vi "V7001 Message Loop.vi"(8 "error in (no error)":errorcluster, 9 "Data Queue":refnum<queue>, 10 "Data Notifier":refnum<notifier>, 11 "Message Queues":T1) -> (0 "error out":errorcluster)   [LabVIEW 2015, in "V7001.lvlib"]
uses:
  V7001.lvlib
  support/Message Queue/All Message Queues.ctl
  support/Message Queue/Message Cluster.ctl
  V7001 Configuration.ctl
  V7001 State.ctl
  V7001 Loop State.ctl
  <vilib>/Utility/error.llb/Error Cluster From Error Code.vi
  <vilib>/ErrorRing/Error Ring.xnode
  support/Message Queue/Message Queue.lvlib
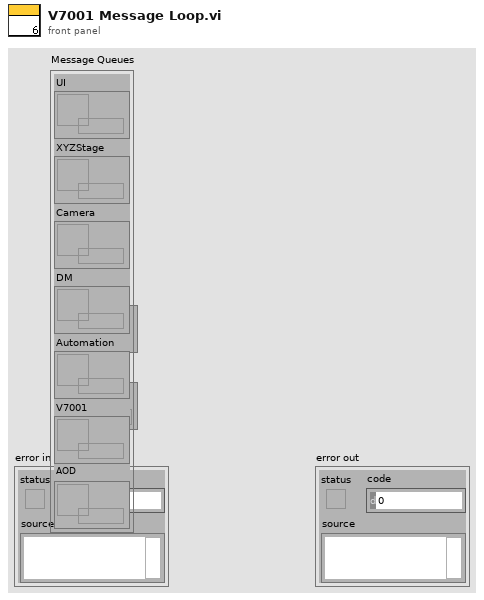
[diagram p1: front panel]
types:
  T1 = typedef "Message Queue.lvlib/All Message Queues.ctl" = cluster{"UI":refnum<queue>, "XYZStage":refnum<queue>, "Camera":refnum<queue>, "DM":refnum<queue>, "Automation":refnum<queue>, "V7001":refnum<queue>, "AOD":refnum<queue>}
  T2 = typedef "V7001.lvlib/V7001 State.ctl" = cluster{"V7001 State":T3, "Handle out":u32, "Size":dbl[]}
  T3 = typedef "V7001.lvlib/V7001 Loop State.ctl" = enum16{"Idle", "Connected"}
  T4 = typedef "V7001.lvlib/V7001 Configuration.ctl" = cluster{" Index":u32}
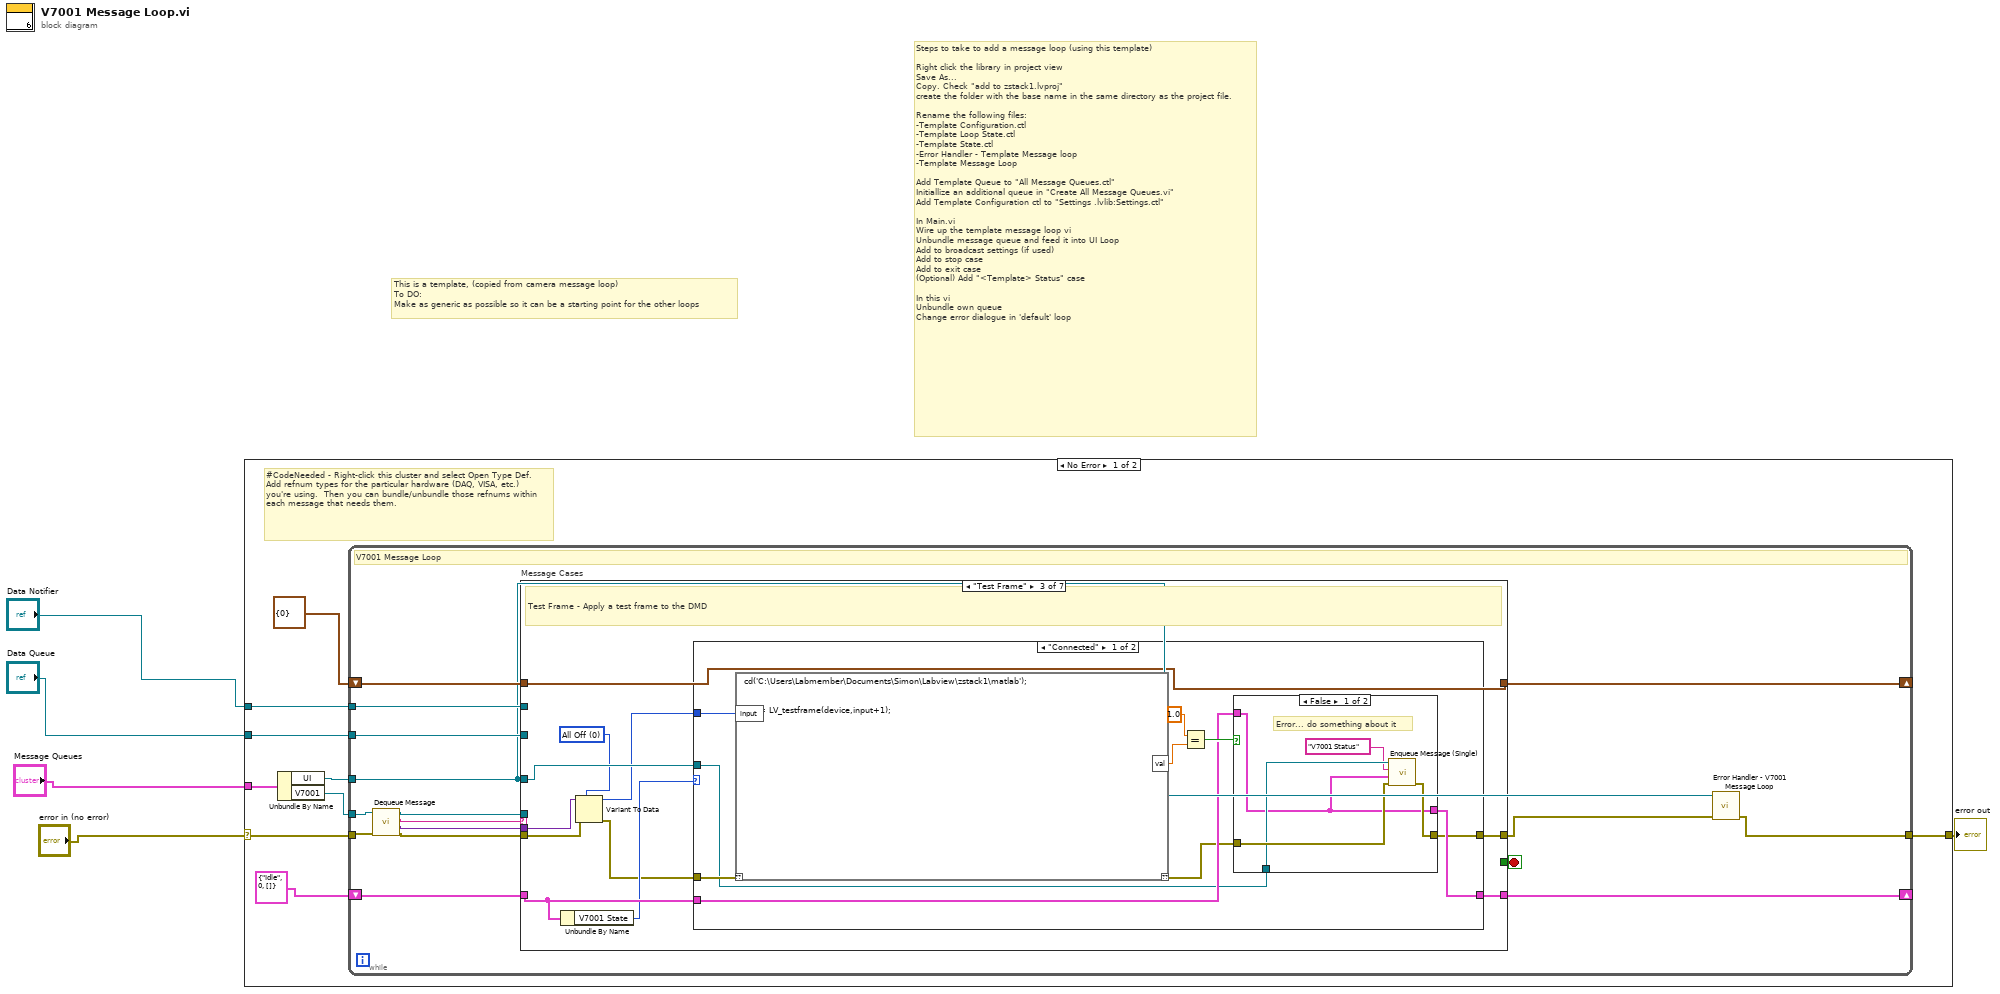
[diagram p0: block diagram]
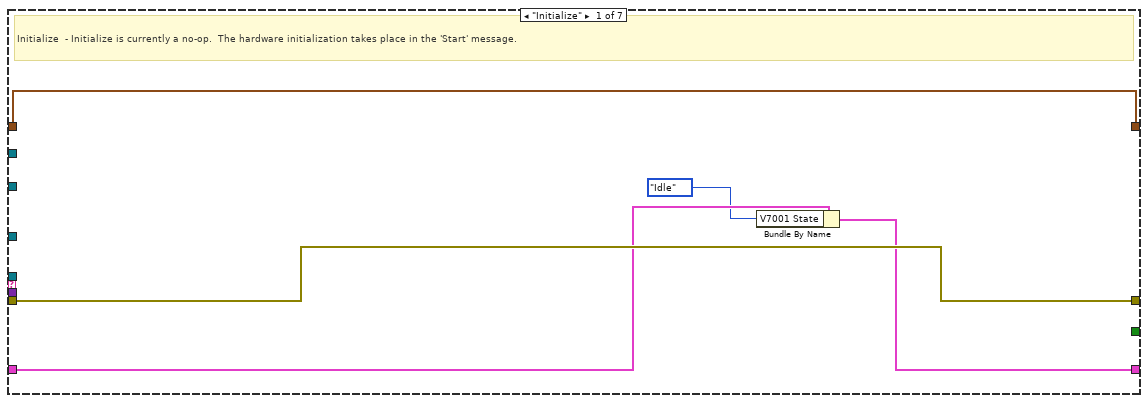
[diagram p2: hidden frame]
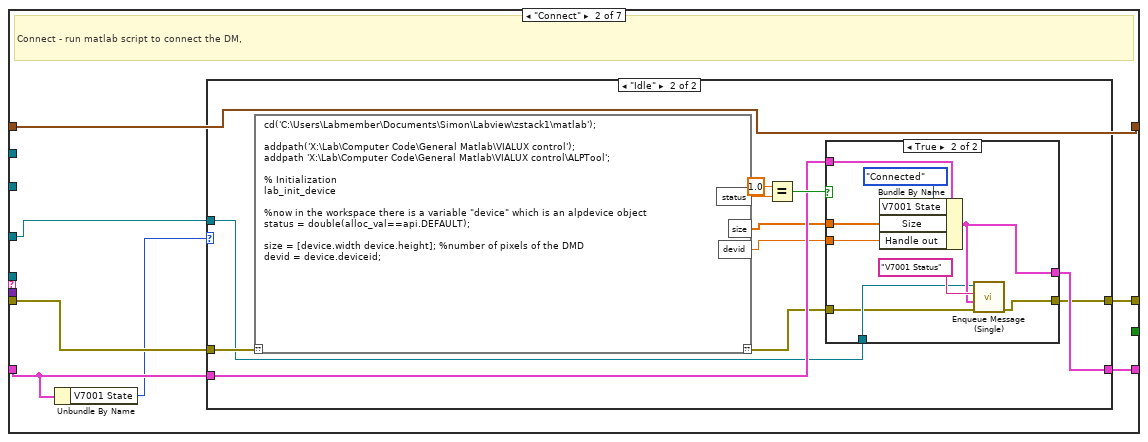
[diagram p3: hidden frame]
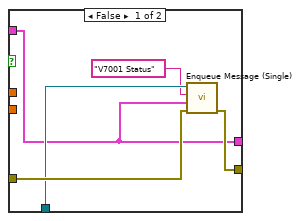
[diagram p5: hidden frame]
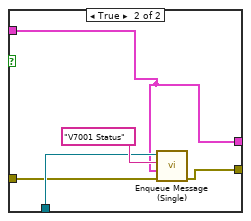
[diagram p6: hidden frame]
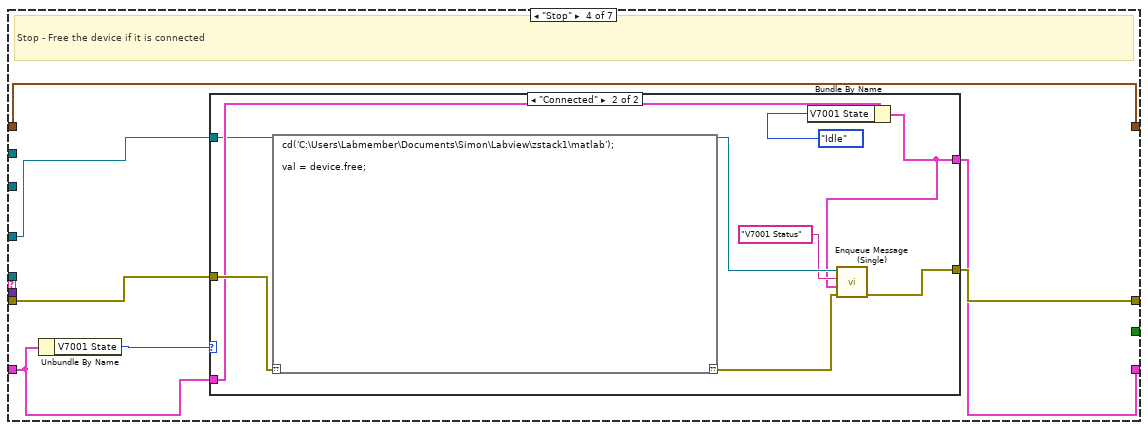
[diagram p8: hidden frame]
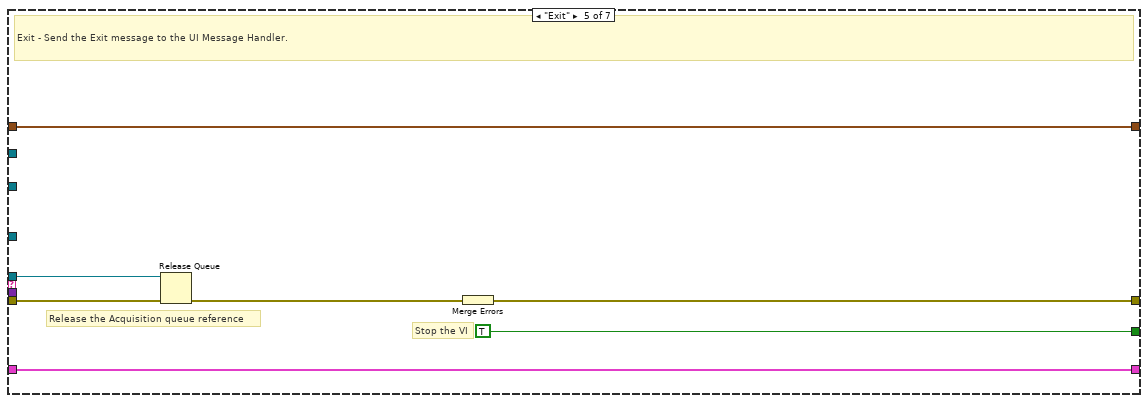
[diagram p10: hidden frame]
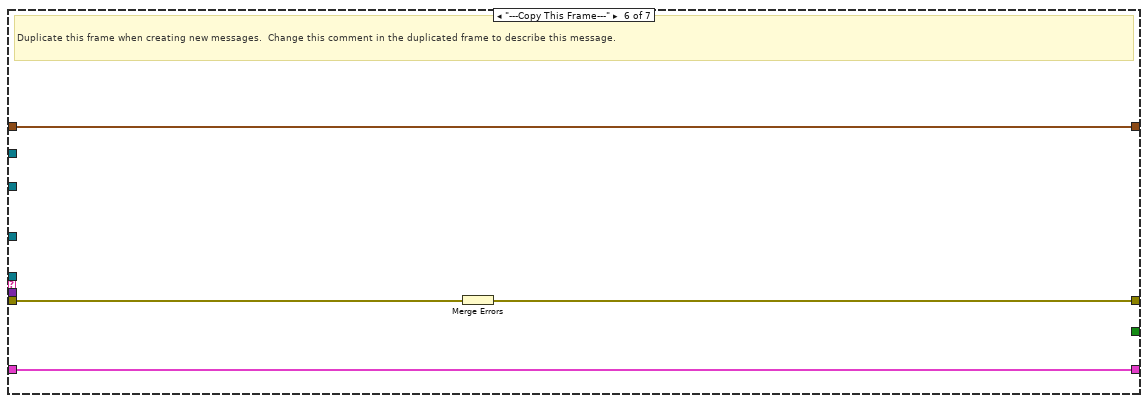
[diagram p11: hidden frame]
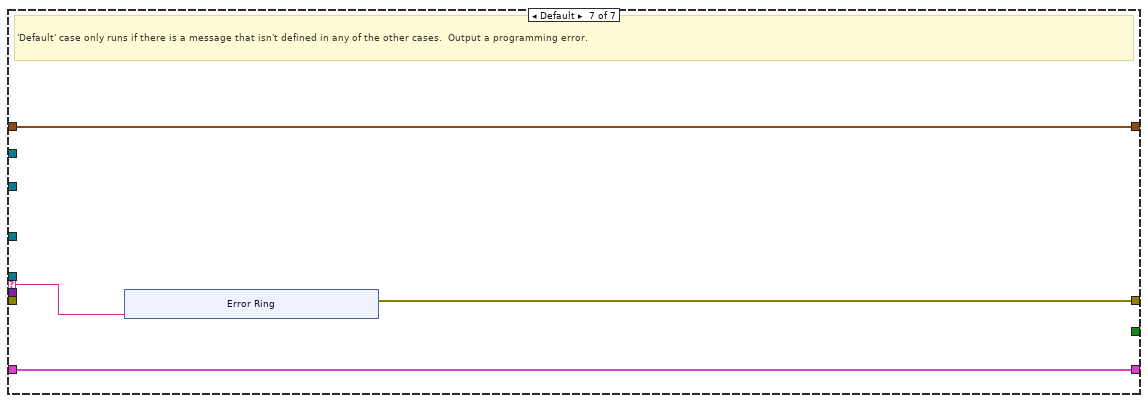
[diagram p12: hidden frame]
diagram:
  # "Steps to take to add a message loop (using this template)\n\nRight click the library in project view\nSave As...\nCopy. Check \"add to zstack1.lvproj\"\ncreate the folder with the base name in the same directory as the project file.\n\nRename the following files:\n-Template Configuration.ctl\n-Template Loop State.ctl\n-Template State.ctl\n-Error Handler - Template Message loop\n-Template Message Loop\n\nAdd Template Queue to \"All Message Queues.ctl\"\nInitiallize an additional queue in \"Create All Message Queues.vi\"\nAdd Template Configuration ctl to \"Settings .lvlib:Settings.ctl\"\n\nIn Main.vi\nWire up the template message loop vi\nUnbundle message queue and feed it into UI Loop\nAdd to broadcast settings (if used)\nAdd to stop case\nAdd to exit case\n(Optional) Add \"<Template> Status\" case\n\nIn this vi\nUnbundle own queue\nChange error dialogue in 'default' loop"
  # "This is a template, (copied from camera message loop)\nTo DO:\nMake as generic as possible so it can be a starting point for the other loops"
  n1 = case shown="No Error" "error in (no error)" {
    selector: "error in (no error)" -> [w11 w142]
    tunnel: "Message Queues" -> [w14 _]
    tunnel: [w12 w142] -> w5
    tunnel: "Data Notifier" -> [w9 _]
    tunnel: "Data Queue" -> [w8 _]
    frame No Error {
      # "#CodeNeeded - Right-click this cluster and select Open Type Def.  Add refnum types for the particular hardware (DAQ, VISA, etc.) you're using.  Then you can bundle/unbundle those refnums within each message that needs them."
      n2 = Unbundle By Name(w14) -> ("UI"=w10:refnum<queue>, "V7001"=w13:refnum<queue>)
      n3 = while {
        tunnel: w13 -> [w23]
        shift-right: [w29] -> _
        shift-left: T4 {" Index"=0} ("Hardware Configuration") -> [w30]
        tunnel: w10 -> [w15]
        tunnel: w9 -> [w27]
        tunnel: w8 -> [w26]
        shift-right: [w24] -> _
        shift-left: T2 {"V7001 State"=enum."Idle", "Handle out"=0, "Size"=[]} ("Cluster") -> [w25]
        tunnel: w11 -> [w22]
        tunnel: [w17] -> w12
        stop <- w28 stop-if-true
        # "V7001 Message Loop"
        n4 = call "Dequeue Message.vi"("error in (no error)"=w22, "Message Queue"=w23) -> ("error out"=w18:errorcluster, "Message Data"=w19:variant, "Message"=w20:string, "dup Message Queue"=w21:refnum<queue>)  [unwired: 6 in]
        n5 = case "Message Cases" shown="\"Test Frame\"" w20 {
          selector: w20 -> [_ _ _ _ _ _ w131]
          tunnel: w21 -> [_ _ _ _ w121 _ _]
          tunnel: w18 -> [w34 w41 w71 w107 w123 w130 _]
          tunnel: [w34 w36 w75 w106 w125 w128 w132] -> w16
          tunnel: w30 -> [w35 w42 w80 w109 w124 w129 w134]
          tunnel: [w35 w42 w80 w109 w124 w129 w134] -> w29
          tunnel: [_ _ _ _ TRUE _ _] -> w28
          tunnel: w19 -> [_ _ w74 _ _ _ _]
          tunnel: w15 -> [_ w37 w76 w103 _ _ _]
          tunnel: w27 -> [_ _ _ _ _ _ _]
          tunnel: w26 -> [_ _ _ _ _ _ _]
          tunnel: w25 -> [w32 w39 w78 w105 w120 w127 w133]
          tunnel: [w33 w40 w79 w104 w120 w127 w133] -> w24
          frame "Initialize" {
            # "Initialize  - Initialize is currently a no-op.  The hardware initialization takes place in the 'Start' message."
            n6 = Bundle By Name(cluster=w32, "V7001 State"=V7001_Loop_State."Idle") -> (w33:T2)
          }
          frame "Connect" {
            # "Connect - run matlab script to connect the DM,"
            n7 = Unbundle By Name(w39) -> ("V7001 State"=w38:T3)
            n8 = case shown="\"Idle\"" w38 {
              tunnel: w41 -> [w44 w55]
              tunnel: w39 -> [w43 w51]
              tunnel: [w43 w50] -> w40
              tunnel: w37 -> [_ w48]
              tunnel: [w44 w46] -> w36
              frame "Connected", Default {
              }
              frame "Idle" {
                n9 = script code="cd('C:\\Users\\Labmember\\Documents\\Simon\\Labview\\zstack1\\matlab');\n\naddpath('X:\\Lab\\Computer Code\\General Matlab\\VIALUX control');\naddpath 'X:\\Lab\\Computer Code\\General Matlab\\VIALUX control\\ALPTool';\n\n% Initialization \nlab_init_device\n\n%now in the workspace there is a variable \"device\" which is an alpdevice object\nstatus = double(alloc_val==api.DEFAULT);\n\nsize = [device.width device.height]; %number of pixels of the DMD\ndevid = device.deviceid;"("??"=w55) -> ("??"=w47:errorcluster, "status"=w54:dbl, "size"=w49:dbl[], "devid"=w45:dbl)
                n10 = Equal?(x=1.0, y=w54) -> (x = y?=w52:bool)
                n11 = case shown="True" w52 {
                  tunnel: [w56 w65] -> w50
                  tunnel: w51 -> [w56 w69]
                  tunnel: w49 -> [_ w67]
                  tunnel: w48 -> [w58 w64]
                  tunnel: w47 -> [w59 w63]
                  tunnel: [w60 w62] -> w46
                  tunnel: w45 -> [_ w61]
                  frame False {
                    n12 = call "Enqueue Message (Single).vi"("error in (no error)"=w59, "Message Data"=w56, "Message"="V7001 Status", "Message Queue"=w58) -> ("error out"=w60:errorcluster)  [unwired: 6 in, 1 out]
                  }
                  frame True {
                    n13 = Bundle By Name(cluster=w69, "V7001 State"=V7001_Loop_State."Connected", "Size"=w67, "Handle out"=w61) -> (w65:T2)
                    n14 = call "Enqueue Message (Single).vi"("error in (no error)"=w63, "Message Data"=w65, "Message"="V7001 Status", "Message Queue"=w64) -> ("error out"=w62:errorcluster)  [unwired: 6 in, 1 out]
                  }
                }
              }
            }
          }
          frame "Test Frame" {
            w73 = u16 0 items=["All Off", "All On", "Checkerboard 1", "Random"] ("Frame")
            # "Test Frame - Apply a test frame to the DMD"
            n15 = Unbundle By Name(w78) -> ("V7001 State"=w77:T3)
            n16 = Variant To Data(error in=w71, type=w73, Variant=w74) -> (data=w72:u16, error out=w70:errorcluster)
            n17 = case shown="\"Connected\"" w77 {
              tunnel: w70 -> [w90 w102]
              tunnel: w78 -> [w86 w101]
              tunnel: [w85 w101] -> w79
              tunnel: w76 -> [w84 _]
              tunnel: [w82 w102] -> w75
              tunnel: w72 -> [w81 _]
              frame "Connected" {
                n18 = script code="cd('C:\\Users\\Labmember\\Documents\\Simon\\Labview\\zstack1\\matlab');\n\n\nval = LV_testframe(device,input+1);"("??"=w90, "input"=w81) -> ("??"=w83:errorcluster, "val"=w89:dbl)
                n19 = Equal?(x=1.0, y=w89) -> (x = y?=w87:bool)
                n20 = case shown="False" w87 {
                  tunnel: [w91 w96] -> w85
                  tunnel: w86 -> [w91 w96]
                  tunnel: w84 -> [w93 w99]
                  tunnel: w83 -> [w94 w98]
                  tunnel: [w95 w97] -> w82
                  frame False {
                    # "Error... do something about it"
                    n21 = call "Enqueue Message (Single).vi"("error in (no error)"=w94, "Message Data"=w91, "Message"="V7001 Status", "Message Queue"=w93) -> ("error out"=w95:errorcluster)  [unwired: 6 in, 1 out]
                  }
                  frame True {
                    n22 = call "Enqueue Message (Single).vi"("error in (no error)"=w98, "Message Data"=w96, "Message"="V7001 Status", "Message Queue"=w99) -> ("error out"=w97:errorcluster)  [unwired: 6 in, 1 out]
                  }
                }
              }
              frame "Idle", Default {
              }
            }
          }
          frame "Stop" {
            # "Stop - Free the device if it is connected"
            n23 = Unbundle By Name(w105) -> ("V7001 State"=w108:T3)
            n24 = case shown="\"Connected\"" w108 {
              tunnel: w107 -> [w110 w119]
              tunnel: [w110 w114] -> w106
              tunnel: [w111 w112] -> w104
              tunnel: w105 -> [w111 w118]
              tunnel: w103 -> [_ w116]
              frame "Idle", Default {
              }
              frame "Connected" {
                n25 = script code="cd('C:\\Users\\Labmember\\Documents\\Simon\\Labview\\zstack1\\matlab');\n\nval = device.free;"("??"=w119) -> ("??"=w115:errorcluster)
                n26 = Bundle By Name(cluster=w118, "V7001 State"=V7001_Loop_State."Idle") -> (w112:T2)
                n27 = call "Enqueue Message (Single).vi"("error in (no error)"=w115, "Message Data"=w112, "Message"="V7001 Status", "Message Queue"=w116) -> ("error out"=w114:errorcluster)  [unwired: 6 in, 1 out]
              }
            }
          }
          frame "Exit" {
            # "Release the Acquisition queue reference"
            # "Stop the VI"
            # "Exit - Send the Exit message to the UI Message Handler."
            n28 = Release Queue(queue=w121, error in (no error)=w123) -> (error out=w122:errorcluster)  [unwired: 1 in, 2 out]
            n29 = Merge Errors(w122) -> (w125:errorcluster)
          }
          frame "---Copy This Frame---" {
            # "Duplicate this frame when creating new messages.  Change this comment in the duplicated frame to describe this message."
            n30 = Merge Errors(w130) -> (w128:errorcluster)
          }
          frame Default {
            # "'Default' case only runs if there is a message that isn't defined in any of the other cases.  Output a programming error."
            n31 = xnode "Error Ring"("parameter 0"=w131) -> ("error out"=w132:errorcluster)
          }
        }
        n32 = call "Error Handler - V7001 Message Loop.vi"("error in (no error)"=w16, "Message Queue"=w15) -> ("dup error in"=w17:errorcluster)  [unwired: 8 in, 1 out]
      }
    }
    frame Error {
    }
  }
  "error out" <- w5
